vi "Database Recordset Set Connnection.vi"(8 "error in (no error)":errorcluster caption="错误输入（无错误）", 10 "Database Connection.lvclass":refnum<class "Database Connection.lvclass">, 11 "Database Recordset 输入":refnum<class "Database Recordset.lvclass"> caption="DNL_LabVIEW Object in") -> (0 "error out":errorcluster caption="错误输出", 3 "Database Recordset 输出":refnum<class "Database Recordset.lvclass"> caption="DNL_LabVIEW Object out")   [LabVIEW 2011, in "Database Recordset.lvclass"]
uses:
  Database Recordset.lvclass
  Connection/Database Connection.lvclass
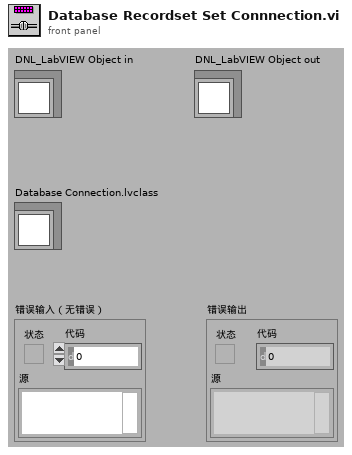
[diagram p1: front panel]
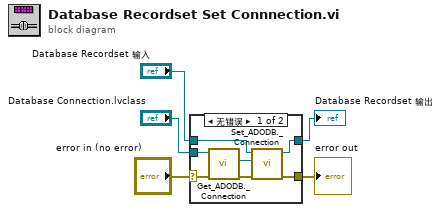
[diagram p0: block diagram]
diagram:
  n1 = case shown="无错误" "error in (no error)" {
    selector: "error in (no error)" -> [w8 w14]
    tunnel: [w6 w14] -> w4
    tunnel: [w11 w13] -> w2
    tunnel: "Database Recordset 输入" -> [w12 w13]
    tunnel: "Database Connection.lvclass" -> [w10 _]
    frame No Error {
      n2 = call "Get_ADODB._Connection.vi"("error in (no error)"=w8, "Database Connection输入"=w10) -> ("error out"=w7:errorcluster, "ADODB._Connection"=w9:refnum<k7>)  [unwired: 7 in, 1 out]
      n3 = call "Set_ADODB._Connection.vi"("error in (no error)"=w7, "ADODB._Connection"=w9, "Database Recordset输入"=w12) -> ("error out"=w6:errorcluster, "Database Recordset输出"=w11:refnum<class "Database Recordset.lvclass">)  [unwired: 7 in]
    }
    frame Error {
    }
  }
  "error out" <- w4
  "Database Recordset 输出" <- w2
